vi "GlobalVariable_CSMModeData.vi"() -> ()   [LabVIEW 2017, in "testcase-CSMNonCSMCallerSupportAPI.lvclass"]
uses:
  testcase-CSMNonCSMCallerSupportAPI.lvclass
  InternalCluster.ctl
panel:
  in  "CSM_Mode_Cluster":T1={"Mode"=enum."Others", "#Nodes"=0}
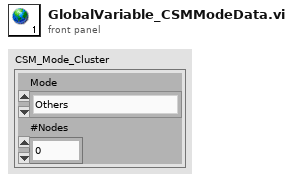
[diagram p1: front panel]
types:
  T1 = typedef "testcase-CSMNonCSMCallerSupportAPI.lvclass/InternalCluster.ctl" = cluster{"Mode":enum16{"Invalid", "Others", "WorkerAgent or Chain"}, "#Nodes":u32}
diagram:
